vi "GymkhanaFlagSign.vi"(9 "GreenFlagSignal":bool, 10 "RedFlagSignal":bool, 11 "inputFlageData":T1) -> (3 "outputFlageData":T1)   [LabVIEW 2020]
uses:
  CommonControl/Flag.ctl
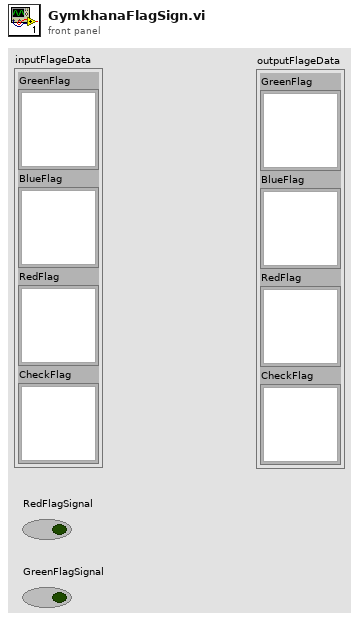
[diagram p1: front panel]
types:
  T1 = typedef "Flag.ctl" = cluster{"GreenFlag":picture, "BlueFlag":picture, "RedFlag":picture, "CheckFlag":picture}
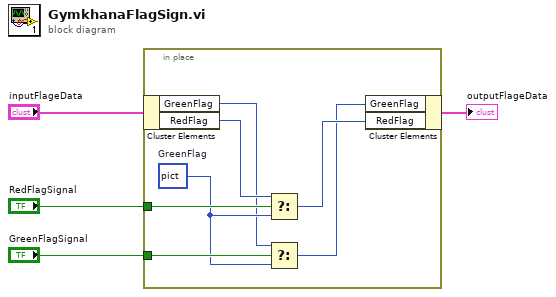
[diagram p0: block diagram]
diagram:
  n1 = in-place {
    in-place-border: "RedFlagSignal" -> [w11]
    in-place-border: "GreenFlagSignal" -> [w10]
    w9 = picture data[5B]  # GreenFlag
    n2 = in-place-cluster #1("inputFlageData") -> ("GreenFlag"=w7:picture, "RedFlag"=w8:picture)
    n3 = Select(t=w8, s=w11, f=w9) -> (s? t:f=w6:picture)
    n4 = Select(t=w7, s=w10, f=w9) -> (s? t:f=w5:picture)
    n5 = in-place-cluster #1("GreenFlag"=w5, "RedFlag"=w6) -> (→"outputFlageData":T1)
  }
